vi "JGPR1.vi"() -> ()   [LabVIEW 2019]
doc: "This Project explores the generation of periodic signals, additive noise, and signal filtering using software based IT filters.\n\nJuan Gamez\nP3600 \nCSUSB Physics"
uses:
  typedefs/periodic signal control.ctl
  <vilib>/ptbypt/NI_PtbyPt.lvlib
panel:
  in  "Tab Control":enum32{"Signal Generation", "Filtering"}(tab)=enum."Filtering"
  in  "combo mode":bool
  in  "Source A":T1={"source"=TRUE, "source type"=FALSE, "Amplitude"=1.0, "Period (steps)"=10.0} {"Amplitude" scale=0.0..1.0; "Period (steps)" scale=1.0..1000.0}
  in  "white noise amplitude":dbl(slide)=0.2 scale=0.0..1.0
  in  "white noise":bool
  in  "Source B":T1={"source"=TRUE, "source type"=FALSE, "Amplitude"=1.0, "Period (steps)"=100.0} {"Amplitude" scale=0.0..1.0; "Period (steps)" scale=1.0..1000.0}
  in  "Low pass":bool=TRUE
  in  "High pass":bool
  in  "LP Corner Period":dbl(slide)=50.0 caption="Low Pass Corner Period (steps)" scale=1.0..1000.0
  in  "HP Corner Period":dbl(slide)=30.0 caption="High Pass Corner Period (steps)" scale=1.0..1000.0
  in  "stop":bool
  in  "update interval (ms)":u32(slide)=20 scale=1.0..1000.0
  out "Waveform Chart":cluster{"Signal out":dbl, "output":dbl}(graph)={"Signal out"=1.635603622223842, "output"=0.29206023666217684}
  # "Signal Generation and Filtering"
  # "Juan Gamez\nP3600\nProject 1"
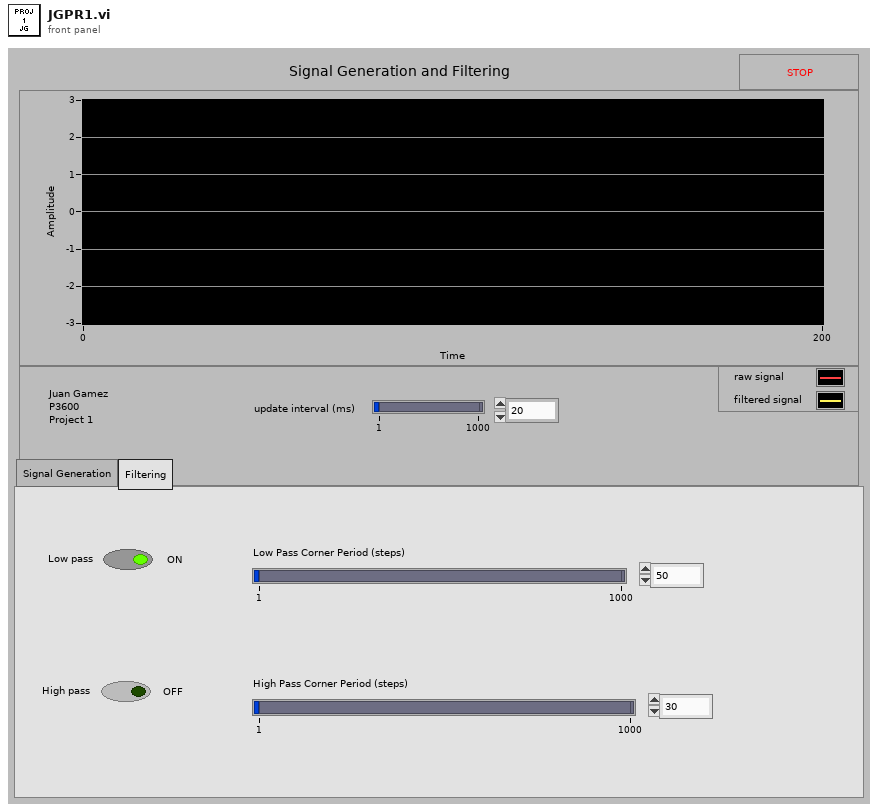
[diagram p1: front panel]
types:
  T1 = typedef "periodic signal control.ctl" = cluster{"source":bool, "source type":bool, "Amplitude":dbl, "Period (steps)":dbl}
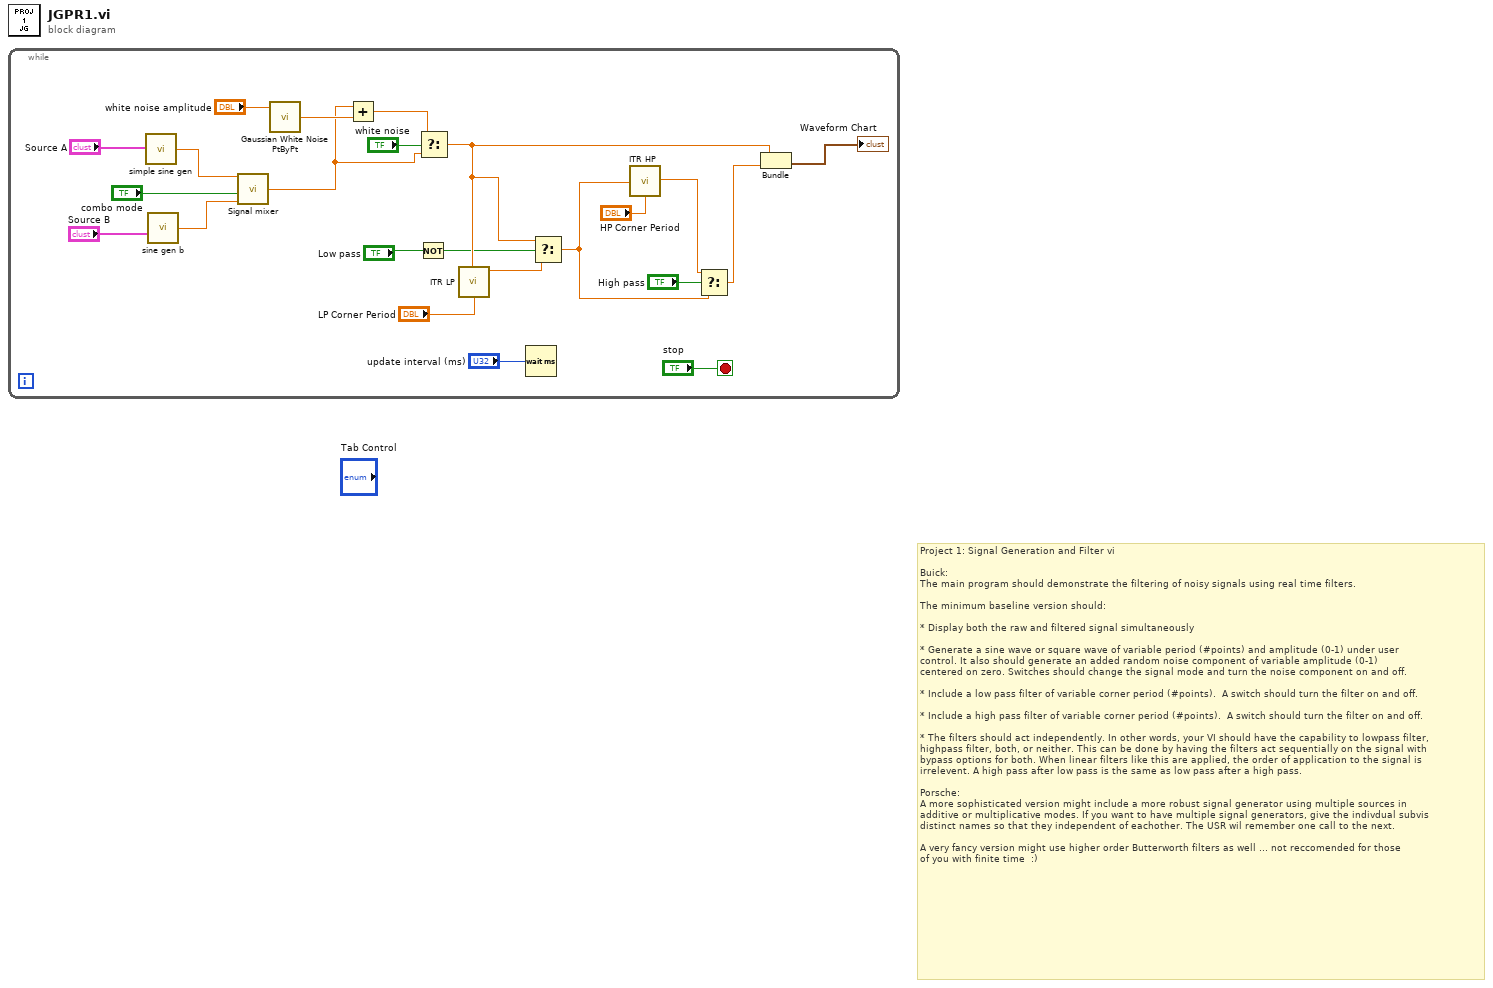
[diagram p0: block diagram]
diagram:
  # "Project 1: Signal Generation and Filter vi\n\nBuick:\nThe main program should demonstrate the filtering of noisy signals using real time filters.\n\nThe minimum baseline version should:\n\n* Display both the raw and filtered signal simultaneously\n\n* Generate a sine wave or square wave of variable period (#points) and amplitude (0-1) under user\ncontrol. It also should generate an added random noise component of variable amplitude (0-1) \ncentered on zero. Switches should change the signal mode and turn the noise component on and off.\n\n* Include a low pass filter of variable corner period (#points).  A switch should turn the filter on and off.\n\n* Include a high pass filter of variable corner period (#points).  A switch should turn the filter on and off.\n\n* The filters should act independently. In other words, your VI should have the capability to lowpass filter,\nhighpass filter, both, or neither. This can be done by having the filters act sequentially on the signal with\nbypass options for both. When linear filters like this are applied, the order of application to the signal is \nirrelevent. A high pass after low pass is the same as low pass after a high pass.\n\nPorsche:\nA more sophisticated version might include a more robust signal generator using multiple sources in \nadditive or multiplicative modes. If you want to have multiple signal generators, give the indivdual subvis \ndistinct names so that they independent of eachother. The USR wil remember one call to the next.\n\nA very fancy version might use higher order Butterworth filters as well ... not reccomended for those\nof you with finite time  :)"
  n1 = while {
    stop <- "stop" stop-if-true
    n2 = call "simple sine gen.vi"("Source"="Source A") -> ("output"=w4:dbl)  [unwired: 14 in]
    n3 = call "sine gen b.vi"("Source"="Source B") -> ("output"=w3:dbl)  [unwired: 14 in]
    n4 = call "Signal mixer.vi"("source A"=w4, "combo mode"="combo mode", "source B"=w3) -> ("output"=w2:dbl)  [unwired: 12 in]
    n5 = call <vilib>:"Gaussian White Noise PtByPt.vi"("standard deviation"="white noise amplitude") -> ("Gaussian white noise"=w19:dbl)  [unwired: 2 in]
    n6 = Add(x=w2, y=w19) -> (x+y=w11:dbl)
    n7 = Not(x="Low pass") -> (.not. x?=w13:bool)
    n8 = Select(t=w11, s="white noise", f=w2) -> (s? t:f=w18:dbl)
    n9 = call "ITR LP.vi"("input"=w18, "corner period (steps)"="LP Corner Period") -> ("output"=w17:dbl)  [unwired: 13 in]
    n10 = Wait (ms)(milliseconds to wait="update interval (ms)") -> ()  [unwired: 1 out]
    n11 = Select(t=w18, s=w13, f=w17) -> (s? t:f=w7:dbl)
    n12 = call "ITR HP.vi"("input"=w7, "corner period (steps)"="HP Corner Period") -> ("output"=w8:dbl)  [unwired: 13 in]
    n13 = Select(t=w8, s="High pass", f=w7) -> (s? t:f=w15:dbl)
    n14 = Bundle("output"=w18, "output"=w15) -> (→"Waveform Chart":cluster{"output":dbl, "output":dbl})  [unwired: 1 in]
  }
